vi "Button Group (Set w Reset).vi"(0 "Button 1":bool=TRUE, 5 "Button 2":bool=TRUE, 7 "Button 3":bool=TRUE, 9 "Button 4":bool=TRUE, 11 "Button 5":bool=TRUE, 12 "Universal Reset":bool=TRUE) -> (4 "Button 1 out":bool=TRUE, 6 "Button 2 out":bool=TRUE, 8 "Button 3 out":bool=TRUE, 10 "Button 4 out":bool=TRUE, 15 "Button 5 out":bool=TRUE)   [LabVIEW 2014]
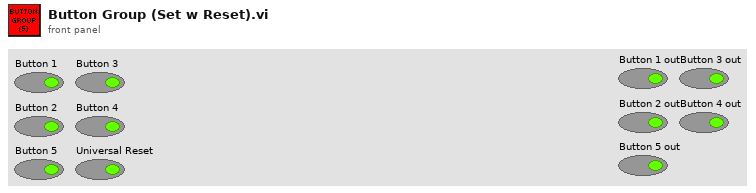
[diagram p1: front panel]
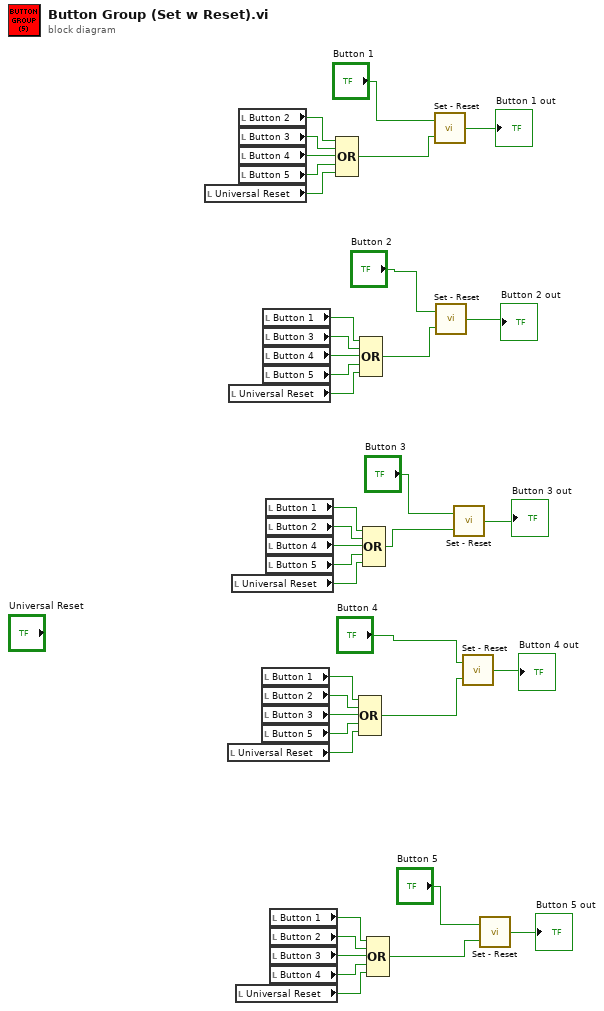
[diagram p0: block diagram]
diagram:
  n1 = local read "Universal Reset"() -> (w36:bool)
  n2 = local read "Universal Reset"() -> (w16:bool)
  n3 = local read "Universal Reset"() -> (w32:bool)
  n4 = local read "Universal Reset"() -> (w20:bool)
  n5 = local read "Universal Reset"() -> (w5:bool)
  n6 = local read "Button 2"() -> (w38:bool)
  n7 = local read "Button 3"() -> (w39:bool)
  n8 = local read "Button 4"() -> (w40:bool)
  n9 = local read "Button 5"() -> (w37:bool)
  n10 = local read "Button 1"() -> (w14:bool)
  n11 = local read "Button 2"() -> (w13:bool)
  n12 = local read "Button 3"() -> (w12:bool)
  n13 = local read "Button 5"() -> (w15:bool)
  n14 = local read "Button 1"() -> (w30:bool)
  n15 = local read "Button 3"() -> (w29:bool)
  n16 = local read "Button 4"() -> (w28:bool)
  n17 = local read "Button 5"() -> (w31:bool)
  n18 = local read "Button 1"() -> (w22:bool)
  n19 = local read "Button 2"() -> (w23:bool)
  n20 = local read "Button 4"() -> (w24:bool)
  n21 = local read "Button 5"() -> (w21:bool)
  n22 = local read "Button 1"() -> (w7:bool)
  n23 = local read "Button 2"() -> (w8:bool)
  n24 = local read "Button 3"() -> (w9:bool)
  n25 = local read "Button 4"() -> (w6:bool)
  n26 = Compound Arithmetic op=OR(w38, w39, w40, w37, w36) -> (w35:bool)
  n27 = Compound Arithmetic op=OR(w14, w13, w12, w15, w16) -> (w11:bool)
  n28 = Compound Arithmetic op=OR(w30, w29, w28, w31, w32) -> (w27:bool)
  n29 = Compound Arithmetic op=OR(w22, w23, w24, w21, w20) -> (w17:bool)
  n30 = Compound Arithmetic op=OR(w7, w8, w9, w6, w5) -> (w4:bool)
  n31 = call "Set - Reset.vi"("Reset"=w35, "Set"="Button 1") -> ("Output"=→"Button 1 out":bool)
  n32 = call "Set - Reset.vi"("Reset"=w27, "Set"="Button 2") -> ("Output"=→"Button 2 out":bool)
  n33 = call "Set - Reset.vi"("Reset"=w17, "Set"="Button 3") -> ("Output"=→"Button 3 out":bool)
  n34 = call "Set - Reset.vi"("Reset"=w11, "Set"="Button 4") -> ("Output"=→"Button 4 out":bool)
  n35 = call "Set - Reset.vi"("Reset"=w4, "Set"="Button 5") -> ("Output"=→"Button 5 out":bool)
